vi "Generate Simulated Data.vi"(8 "error in (no error)":errorcluster, 11 "Signal Type":T1) -> (0 "error out":errorcluster, 2 "Graph Data":waveform(dbl)[](array[waveform]))   [LabVIEW 2018, in "Acquisition.lvlib"]
doc: "Generates sample waveforms according to the signal type in the HW Config input."
uses:
  Acquisition.lvlib
  Signal Type.ctl
  controls/ExitGlobal.vi
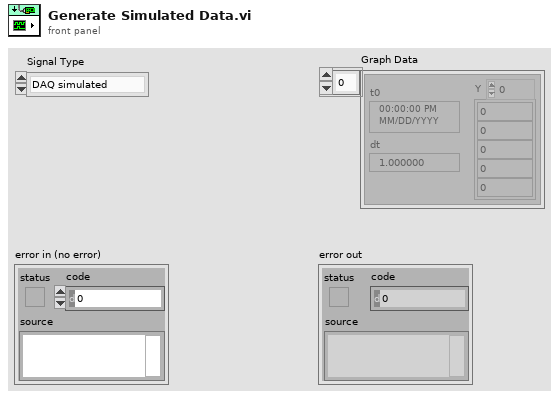
[diagram p1: front panel]
types:
  T1 = typedef "Acquisition.lvlib/Signal Type.ctl" = enum16{"DAQ simulated", "Sine and square wave", "Sine wave"}
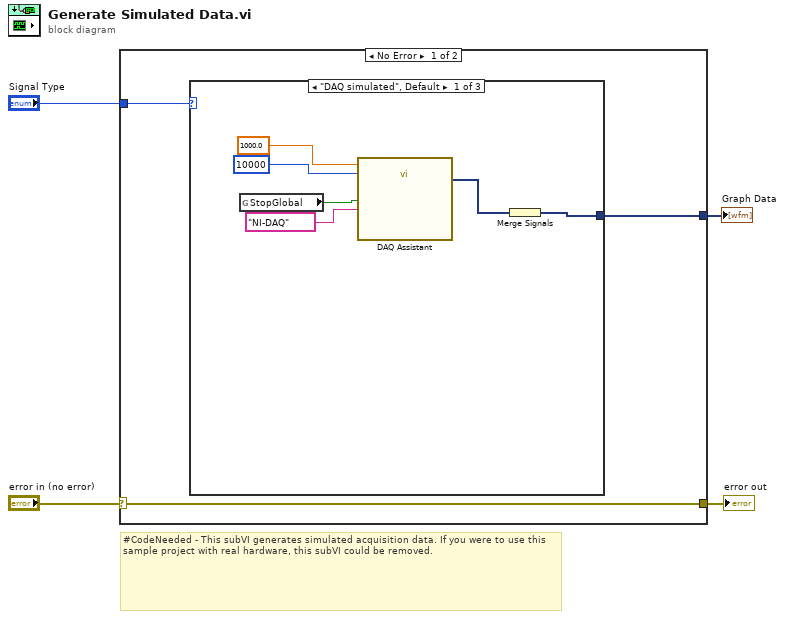
[diagram p0: block diagram]
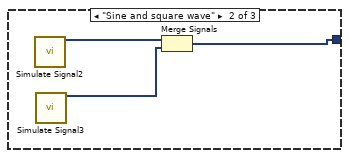
[diagram p2: hidden frame]
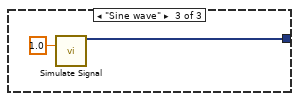
[diagram p3: hidden frame]
diagram:
  # "#CodeNeeded - This subVI generates simulated acquisition data. If you were to use this sample project with real hardware, this subVI could be removed."
  n1 = case shown="No Error" "error in (no error)" {
    selector: "error in (no error)" -> [w7 w19]
    tunnel: [w7 w19] -> w3
    tunnel: [w5 _] -> w2
    tunnel: "Signal Type" -> [w6 _]
    frame No Error {
      n2 = case shown="\"DAQ simulated\", Default" w6 {
        tunnel: [w8 w15 w18] -> w5
        frame "DAQ simulated", Default {
          n3 = global read "ExitGlobal.vi" "StopGlobal"() -> (w11:bool)
          n4 = call "DAQ Assistant"("rate"=1000.0, "number of samples"=10000, "stop (F)"=w11, "device name"=tag "NI-DAQ") -> ("data"=w13:dynamicdata)  [unwired: 12 in, 3 out]
          n5 = Merge Signals(w13) -> (w8:dynamicdata)
        }
        frame "Sine and square wave" {
          n6 = call "Simulate Signal2"() -> ("Square with Gaussian Noise"=w16:dynamicdata)  [unwired: 14 in, 1 out]
          n7 = call "Simulate Signal3"() -> ("Sawtooth with Gaussian Noise"=w14:dynamicdata)  [unwired: 14 in, 1 out]
          n8 = Merge Signals(w16, w14) -> (w15:dynamicdata)
        }
        frame "Sine wave" {
          n9 = call "Simulate Signal"("Frequency"=1.0) -> ("Square with Gaussian Noise"=w18:dynamicdata)  [unwired: 13 in, 1 out]
        }
      }
    }
    frame Error {
    }
  }
  "error out" <- w3
  "Graph Data" <- w2
